vi "tes assemble (fuzzy) edit.vi"() -> ()   [LabVIEW 2015]
uses:
  <vilib>/userdefined/High Color/IMAQdx.ctl
  <vilib>/Platform/TimedLoop/XDataNode/timing_clust.ctl
  <vilib>/Platform/TimedLoop/XDataNode/nitl_modes.ctl
  <vilib>/Platform/TimedLoop/XDataNode/wakeup.ctl
  <vilib>/FPGAPlugInAG/myRIO-1900/niLvFpga_Open_myRIO-1900.vi
  <vilib>/rvi/interface/common/dynamic/niFpgaDynamicAddResources.vi
  <vilib>/addons/Fuzzy Logic/FL Fuzzy Controller (MIMO).vi
  <vilib>/FPGAPlugInAG/Dynamic/niLvFpga_Run_Dynamic.vi
  <vilib>/Utility/error.llb/Error Cluster From Error Code.vi
  <vilib>/rvi/errors/niLvFpgaAdjustHostInterfaceError.vi
  <vilib>/FPGAPlugInAG/Dynamic/niLvFpga_Close_Dynamic.vi
  <vilib>/addons/control/pid/pid.llb/PID (DBL).vi
  <vilib>/Platform/TimedLoop/XDataNode/XDataNode.xnode
  <vilib>/rvi/interface/nirviOpenFPGA/nirviOpenFPGA.xnode
  C/Users/ASUS/Documents/LabVIEW Data/TA/FPGA Bitfiles/FPGAv2_FPGATarget2_Assemble3_FPMe1Auxq6o.lvbitx
  C/Users/ASUS/Documents/LabVIEW Data/Assemble.vi
  <vilib>/rvi/interface/nirviMethod/nirviMethod.xnode
  <vilib>/rvi/interface/nirviReadWriteControl/nirviReadWriteControl.xnode
  <vilib>/rvi/interface/nirviCloseFPGA/nirviCloseFPGA.xnode
  <vilib>/rvi/Arithmetic/AddSubMult/XNode/nirviSatArithmetic.xnode
  <vilib>/rvi/interface/Simulation/niFpgaSimulationCallBeginRW.vi
  <vilib>/Platform/TimedLoop/XDataNode/XDNodeRunTimeDep.lvlib
  <vilib>/vision/driver/NI_Vision_Acquisition_Software.lvlib
  <resource>/objmgr/imaqdx.rc
  <vilib>/addons/control/pid/NI_PID_pid.lvlib
  <vilib>/addons/Fuzzy Logic/NI_Fuzzy_Logic_API.lvlib
  NiFpgaLv.dll
  <vilib>/Instr/_visa.llb/VISA Configure Serial Port (Instr).vi
panel:
  out "Battery percentage":dbl(slide) scale=0.0..100.0
  in  "file path":path=path "c:/captue.jpg"
  out "Distance":dbl
  in  "Capture pict.":bool
  out "video modes":string
  in  "video mode":u32=20
  out "?":T1(plugin-control)
  in  "webcam":T2="cam0"
  out "k.kanan":dbl
  out "k.kiri":dbl
  out "x-y 2":dbl
  out "x+y 2":dbl
  out "percp. 2":dbl
  out "w 2":dbl
  out "percp.":dbl
  out "w":dbl
  out "Velo":i32
  out "Acce":i32
  in  "interval 2":u32=1000
  out "Vel":i32
  out "Acc":i32
  in  "interval":u32=1000
  out "x-y":dbl
  out "x+y":dbl
  out "b":dbl
  out "a":dbl
  out "x = y?":bool
  out "(hi.lo)":u16
  out "Velocity (Counts/Interval) 4":i32
  out "Velocity (Counts/Interval) 3":i32
  out "Velocity (Counts/Interval) 2":i32
  out "Velocity (Counts/Interval)":i32
  out "Acceleration (rps/s) 4":dbl
  out "Acceleration (rps/s) 3":dbl
  out "Acceleration (rps/s) 2":dbl
  out "Acceleration (rps/s)":dbl
  out "frame rate [fps]":dbl
  out "STOP Indicator":bool
  in  "Run/Stop":bool
  out "RC ch3":u32
  out "heading":dbl
  in  "gyro reset":bool=TRUE
  out "heading error":dbl
  out "target bearing":dbl
  out "target distance":dbl
  in  "y target":dbl
  in  "x target":dbl
  out "Acceleration (x)[m/s^2] 2":dbl
  out "Speed (x) [m/s]":dbl
  out "(x) Accelero":dbl
  out "Acceleration (y)[m/s^2]  2":dbl
  out "Speed (y) [m/s]":dbl
  out "(y) Accelero":dbl
  out "Acceleration (z)[m/s^2]  2":dbl
  out "Speed (z) [m/s]":dbl
  out "(z) Accelero":dbl
  out "voltage":dbl
  out "var.RTH":dbl
  out "kec.kanan":dbl
  out "kec.kiri":dbl
  out "kecp.kanan":dbl
  out "kecp.kiri":dbl
  out "var.auto":dbl
  in  "Mode":bool
  in  "RTH":bool
  out "relay 4":bool
  out "relay 3":bool
  out "relay 2":bool
  out "relay1":bool
  out "bocor 2":bool
  out "Water_LVL2":dbl
  out "Water_LVL1":dbl
  out "bocor 1":bool
  out "Arus 4":dbl
  out "Arus 3":dbl
  out "Arus1":dbl
  out "Arus2":dbl
  out "En 8":bool
  out "En 7":bool
  out "En 6":bool
  out "En 5":bool
  out "En 4":bool
  out "En 3":bool
  out "En 2":bool
  out "En 1":bool
  out "Rpm 4":dbl
  out "Rpm 3":dbl
  out "Rpm 2":dbl
  out "Rpm 1":dbl
  out "To":dbl
  out "var. manual":dbl
  out "enc 4":i32
  out "enc 3":i32
  out "enc 2":i32
  out "enc 1":i32
  out "Time On4":dbl format="%.2f"
  out "Time On3":dbl format="%.2f"
  out "Time On2":dbl
  out "y position":dbl
  out "x position":dbl
  out "angle":dbl
  out "Toff":dbl
  out "Time On1":dbl
  out "ultrasonik4":sgl
  out "ultrasonik3":sgl
  out "ultrasonik2":sgl
  out "ultrasonik1":sgl
  out "RC ch2":u32
  out "RC ch1":u32
  out "US 4":u32
  out "US3":u32
  out "US2":u32
  out "US1":u32
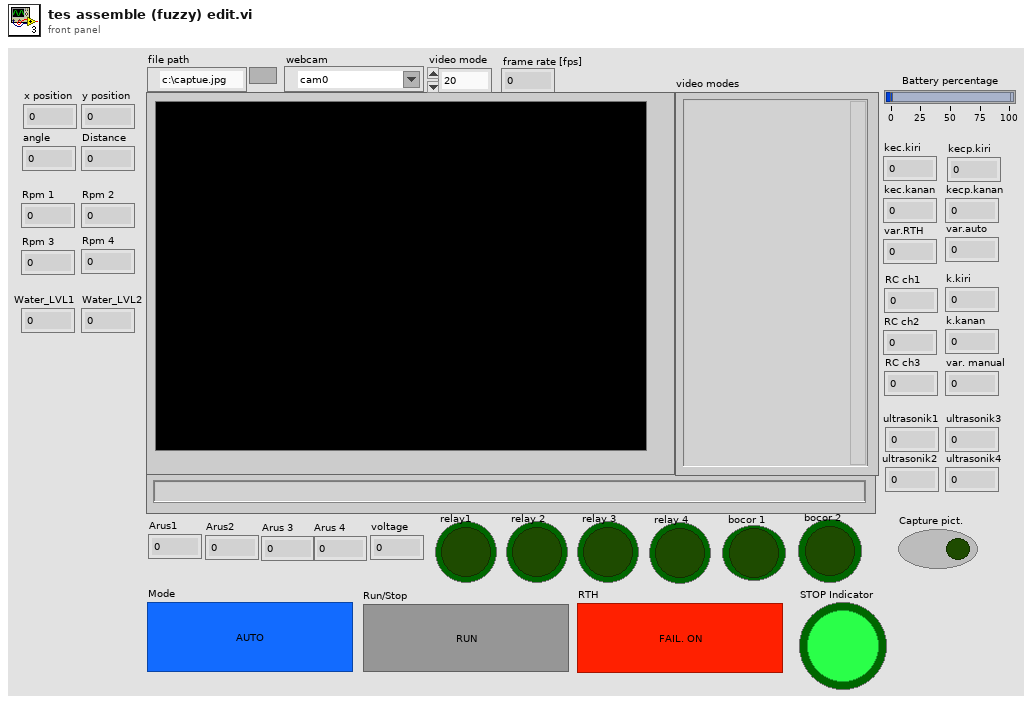
[diagram p1: front panel]
types:
  T1 = typedef "IMAQ Image.ctl" = refnum<image>
  T2 = typedef "IMAQdx.ctl" = refnum<k21>
  T3 = cluster{"Video Mode":u32, "Video Mode Name":string}[]
  T4 = typedef "XDNodeRunTimeDep.lvlib/timing_clust.ctl" = cluster{"Expected End [f-1]":u64, "Actual End [f-1]":u64, "Finished Late? [f-1]":bool, "Expected End [i-1]":u64, "Actual End [i-1]":u64, "Finished Late? [i-1]":bool, "Expected Start [i]":u64, "Actual Start [i]":u64, "Expected Start [f]":u64, "Actual Start [f]":u64, "Source Name":string, "Structure Name":string, "Period":i64, "Deadline":i64, "Offset":i64, "Start":i64, "Priority":i32, "Timeout":i32, "Mode":T5, "Wakeup Reason":T6, "Error":errorcluster, "Source Type":string, "Secondary Source Type":string, "Global End Time":u64, "Global Start Time":u64, "Frame Duration":u64, "Iteration Duration":u64, "Assigned CPU":i32, "I/O Scan Engine Mode":u32}
  T5 = typedef "XDNodeRunTimeDep.lvlib/nitl_modes.ctl" = enum32{"No Change", "Process missed periods, maintain original phase", "Discard missed periods, maintain original phase", "Process missed periods, ignore original phase", "Discard missed periods, ignore original phase"}
  T6 = typedef "XDNodeRunTimeDep.lvlib/wakeup.ctl" = enum32{"Normal", "Aborted", "Asynchronous wakeup", "Timing source error", "Timed loop error", "Timeout"}
  T7 = cluster{"proportional gain (Kc)":dbl, "integral time (Ti, min)":dbl, "derivative time (Td, min)":dbl}
  T8 = typedef "NI_Fuzzy_Logic_API.lvlib/FL System.ctl" = cluster{"input variables":T9[], "output variables":T9[], "rules":T12[], "defuzzification method":T18, "description":string, "user MF interpolating polynomials":T19[]}
  T9 = typedef "NI_Fuzzy_Logic_API.lvlib/FL Variable.ctl" = cluster{"name":string, "range":dbl[], "MFs":T10[]}
  T10 = typedef "NI_Fuzzy_Logic_API.lvlib/FL Membership Function.ctl" = cluster{"name":string, "shape":T11, "points":dbl[], "color":u32, "user-defined shape index":i32}
  T11 = typedef "NI_Fuzzy_Logic_API.lvlib/FL Membership Function Shape.ctl" = u16
  T12 = typedef "NI_Fuzzy_Logic_API.lvlib/FL Rule.ctl" = cluster{"antecedents":T13[], "antecedent connective":T15, "consequents":T16[], "consequent implication":T17, "degree of support":dbl}
  T13 = typedef "NI_Fuzzy_Logic_API.lvlib/FL Antecedent.ctl" = cluster{"Var Index":i32, "MF Index":i32, "Cond":T14}
  T14 = typedef "NI_Fuzzy_Logic_API.lvlib/FL Modifier.ctl" = u16
  T15 = typedef "NI_Fuzzy_Logic_API.lvlib/FL Antecedent Connective.ctl" = u16
  T16 = typedef "NI_Fuzzy_Logic_API.lvlib/FL Consequent.ctl" = cluster{"Var Index":i32, "MF Index":i32, "Cond":T14}
  T17 = typedef "NI_Fuzzy_Logic_API.lvlib/FL Consequent Implication.ctl" = u16
  T18 = typedef "NI_Fuzzy_Logic_API.lvlib/FL Defuzzification.ctl" = u16
  T19 = typedef "NI_Fuzzy_Logic_API.lvlib/FL Interpolating polynomials.ctl" = cluster{"X":dbl[], "Y":dbl[], "Y(x) coeff":dbl[][], "X(y) coeff":dbl[][], "Area(y) coeff":dbl[][], "coa_x(y) coeff":dbl[][]}
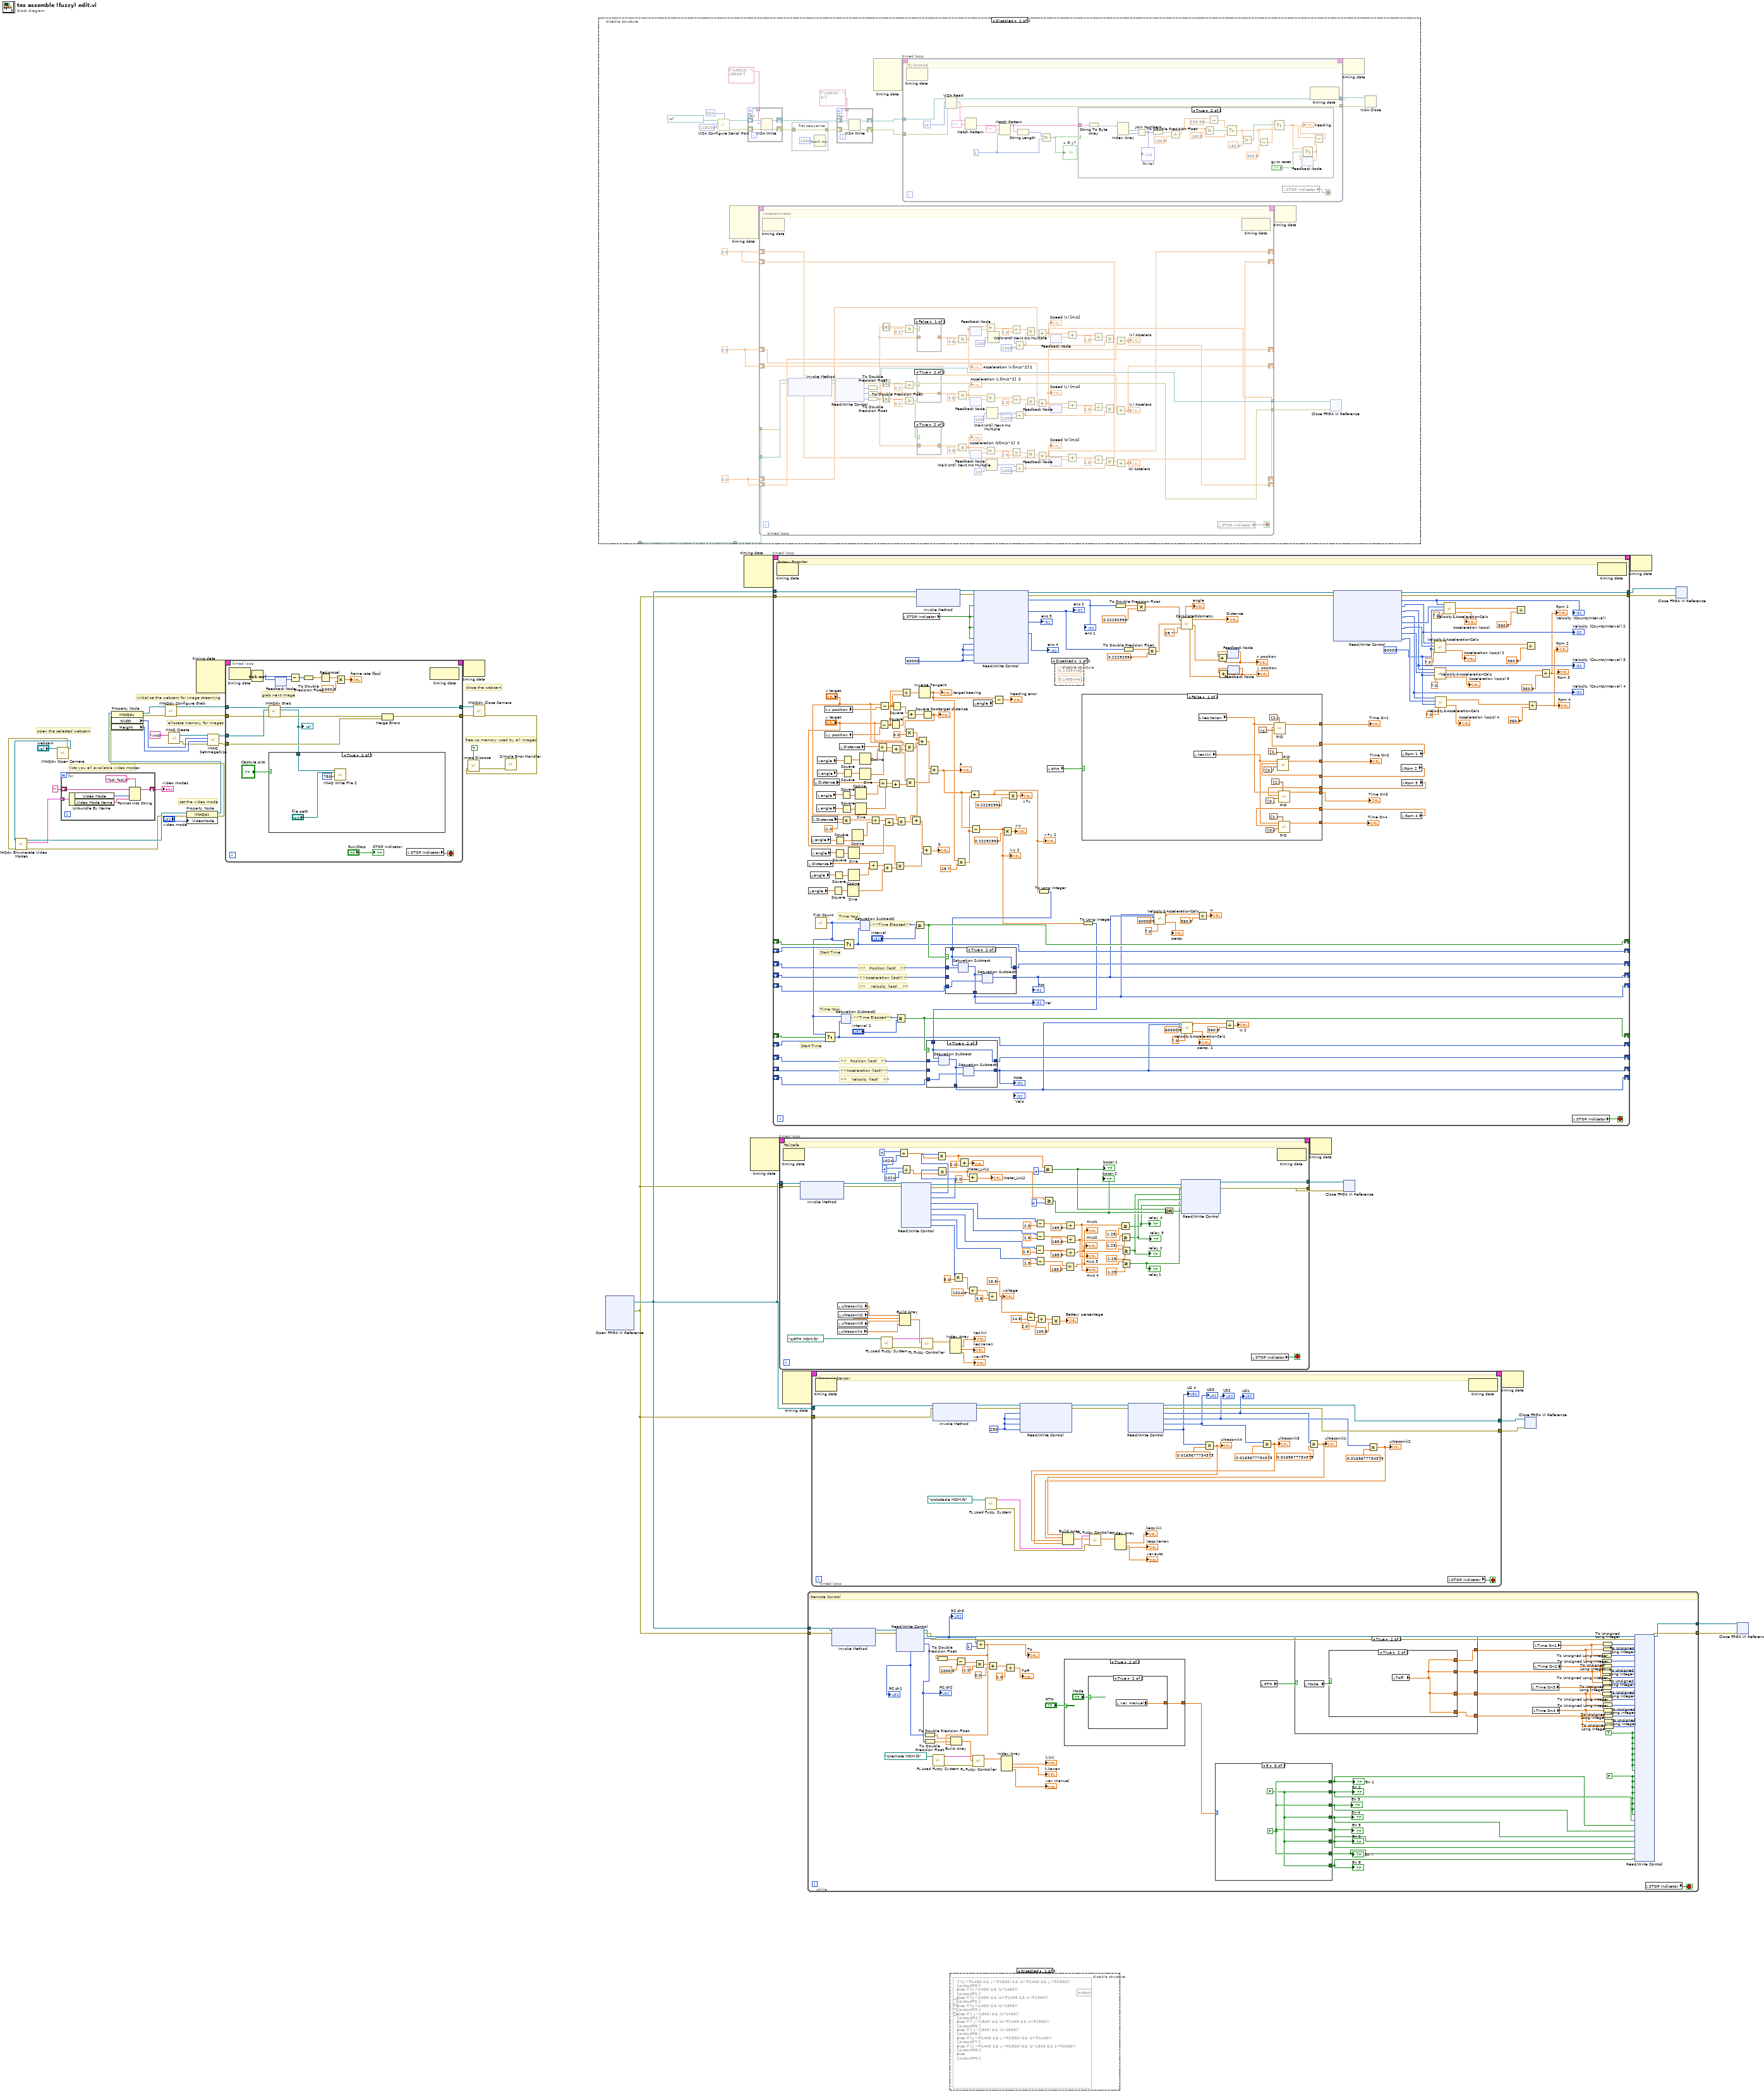
[diagram p0: block diagram]
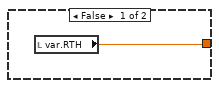
[diagram p4: hidden frame]
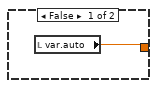
[diagram p5: hidden frame]
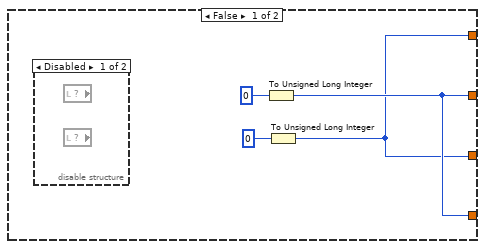
[diagram p6: hidden frame]
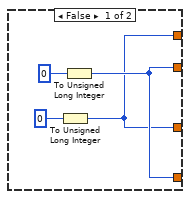
[diagram p8: hidden frame]
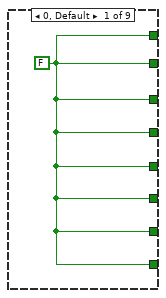
[diagram p9: hidden frame]
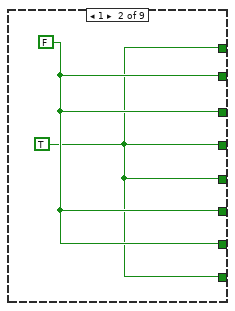
[diagram p10: hidden frame]
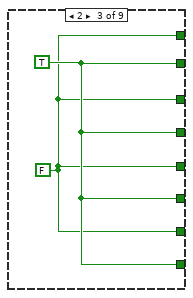
[diagram p11: hidden frame]
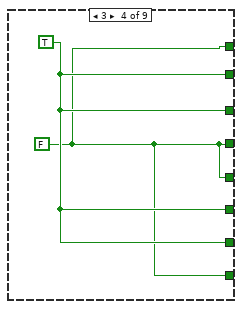
[diagram p12: hidden frame]
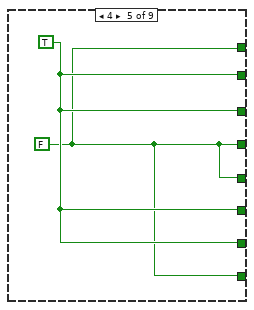
[diagram p13: hidden frame]
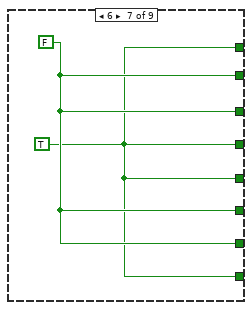
[diagram p14: hidden frame]
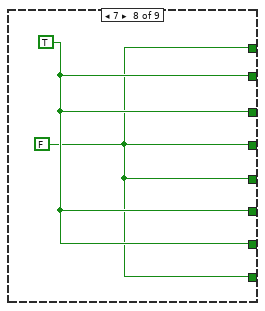
[diagram p15: hidden frame]
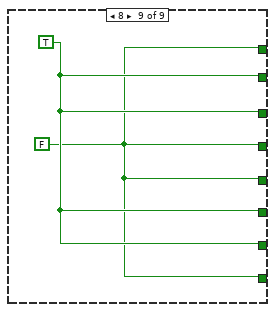
[diagram p16: hidden frame]
diagram:
  # "lists you all available video modes"
  # "close the webcam"
  # "open the selected webcam"
  # "set the video mode"
  # "allocate memory for images"
  # "initialize the webcam for image streaming"
  # "free up memory used by all images"
  n1 = call <vilib>:"IMAQdx Open Camera.vi"("Session In"="webcam") -> ("error out"=w5:errorcluster, "Session Out"=w6:T2)  [unwired: 2 in, 7 out]
  n2 = call <vilib>:"IMAQdx Enumerate Video Modes.vi"("error in"=w5, "Session In"=w6) -> ("error out"=w4:errorcluster, "Video Modes"=w9:T3, "Session Out"=w3:T2)  [unwired: 6 in, 1 out]
  n3 = for {
    tunnel: w9 -> [w51] mode=indexing
    shift-right: [w47] -> w8
    shift-left: "" -> [w46]
    n4 = Unbundle By Name(w51) -> ("Video Mode"=w49:u32, "Video Mode Name"=w48:string)
    n5 = Format Into String(format string="%d: %s\\n", initial string=w46, w49, w48) -> (resulting string=w47:string)  [unwired: 1 in, 1 out]
  }
  "video modes" <- w8
  n6 = call "IMAQ Create"("Image Name"="im0") -> ("New Image"=w19:T1, "error out"=w11:errorcluster)  [unwired: 3 in, 1 out]
  n7 = property on="Property Node" class="IMAQdx"(reference=w3, error in=w4, "VideoMode"="video mode") -> (reference out=w17:T2, error out=w14:errorcluster)
  n8 = property on="Property Node" class="IMAQdx"(reference=w17, error in=w14) -> (reference out=w16:T2, error out=w15:errorcluster, "Width"=w13:u32, "Height"=w12:u32)
  n9 = call <vilib>:"IMAQdx Configure Grab.vi"("error in"=w15, "Session In"=w16) -> ("error out"=w27:errorcluster, "Session Out"=w21:T2)  [unwired: 8 in]
  n10 = node-c288() -> (w2:T4)  [unwired: 4 in]
  n11 = call "IMAQ SetImageSize"("error in (no error)"=w11, "Y Resolution"=w12, "X Resolution"=w13, "Image"=w19) -> ("error out"=w10:errorcluster, "Image Out"=w18:T1)  [unwired: 1 in]
  n12 = timed-loop {
    tunnel: w18 -> [w69]
    tunnel: w27 -> [w67]
    tunnel: w21 -> [w68]
    tunnel: [w64] -> w24
    tunnel: [w65] -> w23
    tunnel: w10 -> [w54]
    timing: w2 -> [_]
    timing-out: [_] -> w1
    stop <- w62 stop-if-true
    # "grab next image"
    n13 = node-c288() -> ()  [unwired: 1 in, 1 out]
    n14 = Tick Count (ms)() -> (millisecond timer value=w61:u32)
    n15 = call <vilib>:"IMAQdx Grab.vi"("error in"=w67, "Image In"=w69, "Session In"=w68) -> ("error out"=w66:errorcluster, "Image Out"=w53:T1, "Session Out"=w65:T2)  [unwired: 5 in, 1 out]
    "?" <- w53
    n16 = case shown="True" "Capture pict." {
      tunnel: w53 -> [_ w72]
      frame False {
      }
      frame True {
        n17 = call-poly "IMAQ Write File 2"("Image Quality"=u32 750, "File Path"="file path", "Image"=w72) -> ()  [unwired: 7 in, 2 out]
      }
    }
    n18 = feedback #1() -> (w60:u32)  [unwired: 1 in]
    n19 = feedback-in #1(w61) -> ()
    n20 = Subtract(x=w61, y=w60) -> (x-y=w59:u32)
    n21 = To Double Precision Float(number=w59) -> (double precision float=w58:dbl)
    n22 = Reciprocal(x=w58) -> (1/x=w57:dbl)
    n23 = Multiply(x=w57, y=1000.0) -> (x*y=→"frame rate [fps]":dbl)
    n24 = Merge Errors(w66, w54) -> (w64:errorcluster)
    n25 = local read "STOP Indicator"() -> (w62:bool)
    n26 = node-c288() -> ()  [unwired: 1 in, 1 out]
    "STOP Indicator" <- "Run/Stop"
  }
  n27 = node-c288(w1) -> ()  [unwired: 1 out]
  n28 = call <vilib>:"IMAQdx Close Camera.vi"("error in"=w24, "Session In"=w23) -> ("error out"=w25:errorcluster)  [unwired: 9 out]
  n29 = call "Imaq Dispose"("All Images? (No)"=TRUE, "error in (no error)"=w25) -> ("error out"=w22:errorcluster)  [unwired: 4 in]
  n30 = call <vilib>:"Simple Error Handler.vi"("error in (no error)"=w22) -> ()  [unwired: 4 in, 5 out]
  n31 = disable-structure shown="Disabled" {
    disable-tunnel: _ -> [w90 _]
    disable-tunnel: _ -> [w89 _]
    frame Disabled {
      w91 = 0.0
      w92 = 0.0
      w93 = 0.0
      n32 = call-poly "VISA Configure Serial Port"("VISA resource name"=refnum<visa-resource-name> "ASRL1::INSTR", "termination char\n(0xA = '\\n' = LF)"=u8 104 ("termination char\n(0xA = '\\n' = LF)"), "baud rate (9600)"=u32 115200) -> ("VISA resource name out"=w87:refnum<visa-resource-name>, "error out"=w85:errorcluster)  [unwired: 11 in]
      n33 = node-c288() -> (w99:T4)  [unwired: 4 in]
      n34 = for {
        shift-right: [w110] -> w81
        shift-left: w87 -> [w111]
        tunnel: string[] ["\u001c", "\u0010"] -> [w109] mode=indexing
        shift-right: [w107] -> w78
        shift-left: w85 -> [w108]
        n35 = VISA Write(VISA resource name=w111, write buffer=w109, error in (no error)=w108) -> (VISA resource name out=w110:refnum<visa-resource-name>, error out=w107:errorcluster)  [unwired: 1 out]
      }
      n36 = timed-loop {
        timing: w99 -> [_]
        timing-out: [_] -> w98
        tunnel: [w234] -> w95
        tunnel: [w233] -> w94
        tunnel: w90 -> [w232]
        tunnel: w89 -> [w231]
        shift-right: [w208] -> _
        shift-left: w93 -> [w218]
        shift-right: [w158] -> _
        shift-left: w93 -> [w209]
        shift-right: [w185] -> _
        shift-left: w92 -> [w189]
        shift-right: [w157] -> _
        shift-left: w92 -> [w188]
        shift-right: [w160] -> _
        shift-left: w91 -> [w164]
        shift-right: [w159] -> _
        shift-left: w91 -> [w163]
        stop <- w156 stop-if-true
        # "Accelerometer"
        n37 = node-c288() -> ()  [unwired: 1 in, 1 out]
        n38 = xnode "Invoke Method"("FPGA VI Reference In"=w232, "error in"=w231) -> ("FPGA VI Reference Out"=w236:refnum<k20>, "error out"=w235:errorcluster)  [unwired: 1 in]
        n39 = xnode "Read/Write Control"("FPGA VI Reference In"=w236, "error in"=w235) -> ("FPGA VI Reference Out"=w234:refnum<k20>, "error out"=w233:errorcluster, "ACC.X.VAL"=w227:u16, "ACC.Y.VAL"=w187:u16, "ACC.Z.VAL"=w162:u16)
        n40 = To Double Precision Float(number=w227) -> (double precision float=w228:dbl)
        n41 = To Double Precision Float(number=w187) -> (double precision float=w186:dbl)
        n42 = To Double Precision Float(number=w162) -> (double precision float=w161:dbl)
        n43 = Absolute Value(x=w228) -> (abs(x)=w229:dbl)
        n44 = Absolute Value(x=w186) -> (abs(x)=w206:dbl)
        n45 = Absolute Value(x=w161) -> (abs(x)=w182:dbl)
        n46 = Greater?(x=w229, y=0.2) -> (0:w230:bool)
        n47 = Greater?(x=w206, y=0.2) -> (0:w207:bool)
        n48 = Greater?(x=w182, y=0.2) -> (0:w183:bool)
        n49 = case shown="False" w230 {
          tunnel: w228 -> [_ w239]
          tunnel: [_ w239] -> w225
          frame False {
          }
          frame True {
          }
        }
        n50 = case shown="True" w207 {
          tunnel: w186 -> [_ w238]
          tunnel: [_ w238] -> w184
          frame False {
          }
          frame True {
          }
        }
        n51 = case shown="True" w183 {
          tunnel: w161 -> [_ w237]
          tunnel: [_ w237] -> w180
          frame False {
          }
          frame True {
          }
        }
        n52 = Multiply(x=w225, y=9.8) -> (x*y=w216:dbl)
        "Acceleration (x)[m/s^2] 2" <- w216
        n53 = Multiply(x=w184, y=9.8) -> (x*y=w196:dbl)
        "Acceleration (y)[m/s^2]  2" <- w196
        n54 = Multiply(x=w180, y=9.8) -> (x*y=w171:dbl)
        "Acceleration (z)[m/s^2]  2" <- w171
        n55 = feedback-in #2(w216) -> ()
        n56 = feedback #2() -> (w217:dbl)  [unwired: 1 in]
        n57 = feedback #3() -> (w197:dbl)  [unwired: 1 in]
        n58 = feedback-in #3(w196) -> ()
        n59 = feedback #4() -> (w172:dbl)  [unwired: 1 in]
        n60 = feedback-in #4(w171) -> ()
        n61 = Add(x=w216, y=w217) -> (x+y=w223:dbl)
        n62 = Add(x=w196, y=w197) -> (x+y=w203:dbl)
        n63 = Add(x=w171, y=w172) -> (x+y=w178:dbl)
        n64 = Wait Until Next ms Multiple(millisecond multiple=10) -> (millisecond timer value=w152:u32)
        n65 = Wait Until Next ms Multiple(millisecond multiple=100) -> (millisecond timer value=w153:u32)
        n66 = Wait Until Next ms Multiple(millisecond multiple=100) -> (millisecond timer value=w154:u32)
        n67 = Divide(x=w223, y=2.0) -> (x/y=w222:dbl)
        n68 = Divide(x=w203, y=2.0) -> (x/y=w202:dbl)
        n69 = Divide(x=w178, y=2.0) -> (x/y=w177:dbl)
        n70 = Divide(x=w154, y=1000) -> (x/y=w211:dbl)
        n71 = Divide(x=w153, y=1000) -> (x/y=w191:dbl)
        n72 = Divide(x=w152, y=1000) -> (x/y=w166:dbl)
        n73 = Multiply(x=w222, y=w211) -> (x*y=w219:dbl)
        n74 = Multiply(x=w202, y=w191) -> (x*y=w198:dbl)
        n75 = Multiply(x=w177, y=w166) -> (x*y=w173:dbl)
        n76 = Add(x=w219, y=w218) -> (x+y=w208:dbl)
        "Speed (x) [m/s]" <- w208
        n77 = Add(x=w198, y=w189) -> (x+y=w185:dbl)
        "Speed (y) [m/s]" <- w185
        n78 = Add(x=w173, y=w164) -> (x+y=w160:dbl)
        "Speed (z) [m/s]" <- w160
        n79 = feedback #5() -> (w215:dbl)  [unwired: 1 in]
        n80 = feedback-in #5(w208) -> ()
        n81 = feedback #6() -> (w195:dbl)  [unwired: 1 in]
        n82 = feedback-in #6(w185) -> ()
        n83 = feedback #7() -> (w170:dbl)  [unwired: 1 in]
        n84 = feedback-in #7(w160) -> ()
        n85 = Add(x=w208, y=w215) -> (x+y=w214:dbl)
        n86 = Add(x=w185, y=w195) -> (x+y=w194:dbl)
        n87 = Add(x=w160, y=w170) -> (x+y=w169:dbl)
        n88 = Divide(x=w214, y=2.0) -> (x/y=w212:dbl)
        n89 = Divide(x=w194, y=2.0) -> (x/y=w192:dbl)
        n90 = Divide(x=w169, y=2.0) -> (x/y=w167:dbl)
        n91 = Multiply(x=w212, y=w211) -> (x*y=w210:dbl)
        n92 = Multiply(x=w192, y=w191) -> (x*y=w190:dbl)
        n93 = Multiply(x=w167, y=w166) -> (x*y=w165:dbl)
        n94 = Add(x=w210, y=w209) -> (x+y=w158:dbl)
        "(x) Accelero" <- w158
        n95 = Add(x=w190, y=w188) -> (x+y=w157:dbl)
        "(y) Accelero" <- w157
        n96 = Add(x=w165, y=w163) -> (x+y=w159:dbl)
        "(z) Accelero" <- w159
        n97 = local read "STOP Indicator"() -> (w156:bool)
        n98 = node-c288() -> ()  [unwired: 1 in, 1 out]
      }
      n99 = flat-sequence {
        tunnel: [w101] -> w79
        tunnel: w78 -> [w101]
        frame #0 {
          n100 = Wait (ms)(milliseconds to wait=u32 1000) -> ()  [unwired: 1 out]
        }
      }
      n101 = for {
        shift-right: [w105] -> w82
        shift-left: w81 -> [w106]
        tunnel: string[] ["\u001b", "\b"] -> [w104] mode=indexing
        shift-right: [w103] -> w83
        shift-left: w79 -> [w102]
        n102 = VISA Write(VISA resource name=w106, write buffer=w104, error in (no error)=w102) -> (VISA resource name out=w105:refnum<visa-resource-name>, error out=w103:errorcluster)  [unwired: 1 out]
      }
      n103 = node-c288() -> (w97:T4)  [unwired: 4 in]
      n104 = timed-loop {
        tunnel: w83 -> [w124]
        tunnel: w82 -> [w125]
        tunnel: [w114] -> w76
        tunnel: [w113] -> w75
        timing: w97 -> [_]
        timing-out: [_] -> w96
        stop <- w112 stop-if-true
        w117 = 1 ("offset (0)")
        # "Gyroscope"
        n105 = node-c288() -> ()  [unwired: 1 in, 1 out]
        n106 = VISA Read(VISA resource name=w125, byte count=u32 14, error in (no error)=w124) -> (VISA resource name out=w114:refnum<visa-resource-name>, read buffer=w122:string, error out=w113:errorcluster)  [unwired: 1 out]
        n107 = Match Pattern(string=w122, regular expression=";") -> (after substring=w120:string)  [unwired: 1 in, 3 out]
        n108 = Match Pattern(string=w120, regular expression=";", offset (0)=w117) -> (before substring=w115:string)  [unwired: 3 out]
        n109 = String Length(string=w115) -> (length=w118:i32)
        n110 = Equal?(x=w118, y=w117) -> (x = y?=w116:bool)
        "x = y?" <- w116
        n111 = case shown="True" w116 {
          tunnel: w115 -> [_ w149]
          frame False {
          }
          frame True {
            n112 = String To Byte Array(string=w149) -> (unsigned byte array=w148:u8[])
            n113 = Index Array(array=w148) -> (element #1=w147:u8, element #2=w146:u8)  [unwired: 2 in]
            n114 = Join Numbers(hi=w147, lo=w146) -> ((hi.lo)=w145:u16)
            "(hi.lo)" <- w145
            n115 = To Double Precision Float(number=w145) -> (double precision float=w144:dbl)
            n116 = Divide(x=w144, y=100.0) -> (x/y=w139:dbl)
            n117 = Greater?(x=w139, y=180.0) -> (0:w142:bool)
            n118 = Subtract(x=w139, y=295.35) -> (x-y=w140:dbl)
            n119 = Select(t=w140, s=w142, f=w139) -> (s? t:f=w134:dbl)
            n120 = Greater?(x=w134, y=180.0) -> (0:w136:bool)
            n121 = Subtract(x=w134, y=360.0) -> (x-y=w135:dbl)
            n122 = Select(t=w135, s=w136, f=w134) -> (s? t:f=w129:dbl)
            n123 = feedback #8() -> (w131:dbl)  [unwired: 1 in]
            n124 = Select(t=w129, s="gyro reset", f=w131) -> (s? t:f=w130:dbl)
            n125 = feedback-in #8(w130) -> ()
            n126 = Subtract(x=w129, y=w130) -> (x-y=→"heading":dbl)
          }
        }
        n127 = local read "STOP Indicator"() -> (w112:bool)
        n128 = node-c288() -> ()  [unwired: 1 in, 1 out]
      }
      n129 = node-c288(w98) -> ()  [unwired: 1 out]
      n130 = xnode "Close FPGA VI Reference"("FPGA VI Reference In"=w95, "error in"=w94) -> ()  [unwired: 1 out]
      n131 = node-c288(w96) -> ()  [unwired: 1 out]
      n132 = VISA Close(VISA resource name=w76, error in (no error)=w75) -> ()  [unwired: 1 out]
    }
    frame Enabled {
    }
  }
  n133 = xnode "Open FPGA VI Reference"() -> ("FPGA VI Reference Out"=w31:refnum<k20>, "error out"=w30:errorcluster)  [unwired: 2 in]
  n134 = node-c288() -> (w39:T4)  [unwired: 4 in]
  n135 = node-c288() -> (w35:T4)  [unwired: 4 in]
  n136 = timed-loop {
    timing: w39 -> [_]
    timing-out: [_] -> w38
    tunnel: w31 -> [w416]
    tunnel: w30 -> [w415]
    tunnel: [w409] -> w37
    tunnel: [w408] -> w36
    shift-right: [w302] -> _
    shift-left: _ -> [w307]
    shift-right: [w301] -> _
    shift-left: _ -> [w306]
    shift-right: [w300] -> _
    shift-left: _ -> [w305]
    shift-right: [w277] -> _
    shift-left: _ -> [w304]
    shift-right: [w278] -> _
    shift-left: _ -> [w303]
    shift-right: [w289] -> _
    shift-left: _ -> [w290]
    shift-right: [w288] -> _
    shift-left: _ -> [w291]
    shift-right: [w287] -> _
    shift-left: _ -> [w292]
    shift-right: [w269] -> _
    shift-left: _ -> [w293]
    shift-right: [w270] -> _
    shift-left: _ -> [w294]
    stop <- w414 stop-if-true
    w372 = u32 60000 ("Velocity Interval (uSec) 4")
    w373 = u32 60000 ("Velocity Interval (uSec) 4")
    # ">>Acceleration (last)>>"
    # "Start Time"
    # ">>    Velocity (last)    >>"
    # ">>   Position (last)   >>"
    # "Time Now"
    # ">>Time Elapsed>>"
    # ">>Acceleration (last)>>"
    # "Start Time"
    # ">>    Velocity (last)    >>"
    # ">>   Position (last)   >>"
    # "Time Now"
    # ">>Time Elapsed>>"
    # "Rotary Encoder"
    n137 = node-c288() -> ()  [unwired: 1 in, 1 out]
    n138 = local read "Distance"() -> (w257:dbl)
    n139 = local read "angle"() -> (w325:dbl)
    n140 = local read "angle"() -> (w330:dbl)
    n141 = local read "angle"() -> (w339:dbl)
    n142 = local read "angle"() -> (w335:dbl)
    n143 = local read "Distance"() -> (w258:dbl)
    n144 = local read "Distance"() -> (w259:dbl)
    n145 = call "Tick Count"() -> ("Tick Count(uSec)"=w295:u32)
    n146 = local read "angle"() -> (w356:dbl)
    n147 = local read "angle"() -> (w352:dbl)
    n148 = local read "angle"() -> (w363:dbl)
    n149 = local read "angle"() -> (w360:dbl)
    n150 = Select(t=w295, s=w290, f=w291) -> (s? t:f=w288:u32)
    n151 = local read "x position"() -> (w398:dbl)
    n152 = local read "y position"() -> (w397:dbl)
    n153 = Square(x=w325) -> (x^2=w326:dbl)
    n154 = Square(x=w330) -> (x^2=w329:dbl)
    n155 = Square(x=w335) -> (x^2=w336:dbl)
    n156 = Square(x=w339) -> (x^2=w340:dbl)
    n157 = local read "Distance"() -> (w260:dbl)
    n158 = Square(x=w356) -> (x^2=w355:dbl)
    n159 = Multiply(x=w258, y=-1.0) -> (x*y=w341:dbl)
    n160 = Square(x=w352) -> (x^2=w351:dbl)
    n161 = xnode ("Saturation Subtract2")("x"=w295, "y"=w288) -> ("x-y"=w296:u32)
    n162 = Square(x=w363) -> (x^2=w362:dbl)
    n163 = Square(x=w360) -> (x^2=w359:dbl)
    n164 = Select(t=w295, s=w307, f=w306) -> (s? t:f=w301:u32)
    n165 = Sine(x=w326) -> (sin(x)=w327:dbl)
    n166 = Cosine(x=w329) -> (cos(x)=w328:dbl)
    n167 = Sine(x=w336) -> (sin(x)=w334:dbl)
    n168 = Cosine(x=w340) -> (cos(x)=w338:dbl)
    n169 = Cosine(x=w355) -> (cos(x)=w354:dbl)
    n170 = Sine(x=w351) -> (sin(x)=w350:dbl)
    n171 = Cosine(x=w362) -> (cos(x)=w361:dbl)
    n172 = Sine(x=w359) -> (sin(x)=w358:dbl)
    n173 = xnode ("Saturation Subtract2")("x"=w295, "y"=w301) -> ("x-y"=w308:u32)
    n174 = Divide(x=w257, y=w328) -> (x/y=w331:dbl)
    n175 = Divide(x=w341, y=w338) -> (x/y=w337:dbl)
    n176 = Divide(x=w260, y=w361) -> (x/y=w357:dbl)
    n177 = Divide(x=w259, y=w354) -> (x/y=w353:dbl)
    n178 = Subtract(x="y target", y=w397) -> (x-y=w396:dbl)
    n179 = Subtract(x="x target", y=w398) -> (x-y=w395:dbl)
    n180 = Add(x=w331, y=w327) -> (x+y=w324:dbl)
    n181 = Add(x=w337, y=w334) -> (x+y=w333:dbl)
    n182 = Square(x=w396) -> (x^2=w400:dbl)
    n183 = Add(x=w353, y=w350) -> (x+y=w348:dbl)
    n184 = Add(x=w357, y=w358) -> (x+y=w349:dbl)
    n185 = Square(x=w395) -> (x^2=w401:dbl)
    n186 = Multiply(x="y target", y=w324) -> (x*y=w319:dbl)
    n187 = Greater Or Equal?(x=w296, y="interval 2") -> (x >= y?=w289:bool)
    n188 = Multiply(x="x target", y=w333) -> (x*y=w322:dbl)
    n189 = Divide(x=w396, y=w395) -> (x/y=w394:dbl)
    n190 = local read "STOP Indicator"() -> (w265:bool)
    n191 = Multiply(x="x target", y=w349) -> (x*y=w345:dbl)
    n192 = Multiply(x="y target", y=w348) -> (x*y=w343:dbl)
    n193 = Add(x=w401, y=w400) -> (x+y=w399:dbl)
    n194 = Greater Or Equal?(x=w308, y="interval") -> (x >= y?=w302:bool)
    n195 = xnode "Invoke Method"("FPGA VI Reference In"=w416, "error in"=w415) -> ("FPGA VI Reference Out"=w418:refnum<k20>, "error out"=w417:errorcluster)  [unwired: 1 in]
    n196 = Inverse Tangent(1:w394) -> (0:w314:dbl)
    "target bearing" <- w314
    n197 = Square Root(x=w399) -> (sqrt(x)=w346:dbl)
    "target distance" <- w346
    n198 = Multiply(x=w346, y=0.0) -> (x*y=w321:dbl)
    n199 = Add(x=w321, y=w322) -> (x+y=w320:dbl)
    n200 = Add(x=w321, y=w345) -> (x+y=w344:dbl)
    n201 = Add(x=w320, y=w319) -> (x+y=→"b":dbl)
    n202 = Add(x=w344, y=w343) -> (x+y=w316:dbl)
    "a" <- w316
    n203 = Multiply(x=w314, y=25.7) -> (x*y=w315:dbl)
    n204 = Add(x=w316, y=w315) -> (x+y=w299:dbl)
    "x+y 2" <- w299
    n205 = Subtract(x=w316, y=w315) -> (x-y=w285:dbl)
    "x-y 2" <- w285
    n206 = local read "angle"() -> (w392:dbl)
    n207 = xnode "Read/Write Control"("FPGA VI Reference In"=w418, "error in"=w417, "Position Reset"=w265, "Position Reset 2"=w265, "Position Reset 3"=w265, "Position Reset 4"=w265, "Velocity Interval (uSec)"=w373, "Velocity Interval (uSec) 2"=w373, "Velocity Interval (uSec) 3"=w373, "Velocity Interval (uSec) 4"=w373) -> ("FPGA VI Reference Out"=w407:refnum<k20>, "error out"=w406:errorcluster, "Position 1"=w250:i32, "Position 2"=w249:i32, "Position 3"=→"enc 3":i32, "Position 4"=→"enc 4":i32)
    "enc 1" <- w250
    "enc 2" <- w249
    n208 = Subtract(x=w314, y=w392) -> (x-y=→"heading error":dbl)
    n209 = Multiply(x=w285, y=0.22292994) -> (x*y=→"x-y":dbl)
    n210 = Multiply(x=w299, y=0.22292994) -> (x*y=→"x+y":dbl)
    n211 = To Long Integer(number=w299) -> (32bit integer=w298:i32)
    n212 = case shown="True" w302 {
      tunnel: w298 -> [_ w486]
      tunnel: w305 -> [w483 w490]
      tunnel: [w485 w489] -> w278
      tunnel: w303 -> [w485 w488]
      tunnel: [w484 w487] -> w277
      tunnel: w304 -> [w484 _]
      tunnel: [w483 w486] -> w300
      frame False {
      }
      frame True {
        n213 = xnode ("Saturation Subtract")("x"=w486, "y"=w490) -> ("x-y"=w489:i32)
        n214 = xnode ("Saturation Subtract3")("x"=w489, "y"=w488) -> ("x-y"=w487:i32)
      }
    }
    "Acc" <- w277
    "Vel" <- w278
    n215 = local read "RTH"() -> (w402:bool)
    n216 = disable-structure shown="Disabled" {
      frame Disabled {
        (unwired) 0.14854461 ("y")
        (unwired) 0.14854461 ("y")
      }
      frame Enabled {
      }
    }
    n217 = To Long Integer(number=w285) -> (32bit integer=w286:i32)
    n218 = case shown="True" w289 {
      tunnel: w286 -> [_ w432]
      tunnel: w292 -> [w429 w436]
      tunnel: [w431 w435] -> w270
      tunnel: w294 -> [w431 w434]
      tunnel: [w430 w433] -> w269
      tunnel: w293 -> [w430 _]
      tunnel: [w429 w432] -> w287
      frame False {
      }
      frame True {
        n219 = xnode ("Saturation Subtract")("x"=w432, "y"=w436) -> ("x-y"=w435:i32)
        n220 = xnode ("Saturation Subtract3")("x"=w435, "y"=w434) -> ("x-y"=w433:i32)
      }
    }
    "Acce" <- w269
    n221 = To Double Precision Float(number=w250) -> (double precision float=w413:dbl)
    n222 = To Double Precision Float(number=w249) -> (double precision float=w412:dbl)
    n223 = Multiply(x=w413, y=0.22292994) -> (x*y=w264:dbl)
    n224 = Multiply(x=w412, y=0.22292994) -> (x*y=w263:dbl)
    n225 = call "Velocity&AccelerationCalc.vi"("Pulses/Revolution"=7.0 ("y"), "Fixed Time \nInterval (uSec)"=60000.0 ("Fixed Time \nInterval (uSec)"), "Acceleration (Counts/Interval)"=w277, "Velocity (Counts/Interval)"=w278) -> ("Acceleration (rps/s)"=→"percp.":dbl, "Velocity (RPM)"=w281:dbl)
    n226 = call "CalculateOdometry.vi"("Left Wheel Distance"=w264, "Right Wheel Distance"=w263, "Wheel Base"=25.7) -> ("output variable"=→"angle":dbl, "Distance"=→"Distance":dbl, "X"=w252:dbl, "Y"=w251:dbl)  [unwired: 2 out]
    n227 = call "Velocity&AccelerationCalc.vi"("Pulses/Revolution"=7.0 ("y"), "Fixed Time \nInterval (uSec)"=60000.0 ("Fixed Time \nInterval (uSec)"), "Acceleration (Counts/Interval)"=w269, "Velocity (Counts/Interval)"=w270) -> ("Acceleration (rps/s)"=→"percp. 2":dbl, "Velocity (RPM)"=w273:dbl)
    n228 = Divide(x=w281, y=360.0) -> (x/y=→"w":dbl)
    n229 = Divide(x=w273, y=360.0) -> (x/y=→"w 2":dbl)
    n230 = feedback #9() -> (w255:dbl)  [unwired: 1 in]
    n231 = Add(x=w255, y=w252) -> (x+y=w254:dbl)
    "x position" <- w254
    n232 = feedback-in #9(w254) -> ()
    n233 = feedback #10() -> (w256:dbl)  [unwired: 1 in]
    n234 = Add(x=w256, y=w251) -> (x+y=w253:dbl)
    "y position" <- w253
    n235 = feedback-in #10(w253) -> ()
    n236 = xnode "Read/Write Control"("FPGA VI Reference In"=w407, "error in"=w406) -> ("FPGA VI Reference Out"=w409:refnum<k20>, "error out"=w408:errorcluster, "Velocity (Counts/Interval)"=w267:i32, "Velocity (Counts/Interval) 2"=w383:i32, "Velocity (Counts/Interval) 3"=w382:i32, "Velocity (Counts/Interval) 4"=w381:i32, "Acceleration (Counts/Interval)"=w391:i32, "Acceleration (Counts/Interval) 2"=w389:i32, "Acceleration (Counts/Interval) 3"=w388:i32, "Acceleration (Counts/Interval) 4"=w387:i32)
    "Velocity (Counts/Interval)" <- w267
    "Velocity (Counts/Interval) 2" <- w383
    "Velocity (Counts/Interval) 3" <- w382
    "Velocity (Counts/Interval) 4" <- w381
    n237 = local read "Rpm 2"() -> (w374:dbl)
    n238 = local read "Rpm 4"() -> (w376:dbl)
    n239 = local read "Rpm 1"() -> (w266:dbl)
    n240 = local read "Rpm 3"() -> (w375:dbl)
    n241 = case shown="False" w402 {
      tunnel: w266 -> [w535 w560]
      tunnel: [w536 w559] -> w268
      tunnel: [w534 w556] -> w405
      tunnel: w374 -> [w533 w555]
      tunnel: w375 -> [w532 w552]
      tunnel: [w531 w551] -> w404
      tunnel: [w529 w548] -> w403
      tunnel: w376 -> [w530 w547]
      frame False {
        n242 = local read "kec.kiri"() -> (w528:dbl)
        n243 = local read "kec.kanan"() -> (w527:dbl)
        n244 = call-poly <vilib>:"PID.vi"("output range"=cluster{"output high":dbl, "output low":dbl} {"output high"=2000.0, "output low"=0.0}, "PID gains"=T7 {"proportional gain (Kc)"=0.3, "integral time (Ti, min)"=0.75, "derivative time (Td, min)"=0.1875}, "process variable"=w535, "setpoint"=w527) -> ("output"=w536:dbl)  [unwired: 6 in, 1 out]
        n245 = call-poly <vilib>:"PID.vi"("output range"=cluster{"output high":dbl, "output low":dbl} {"output high"=2000.0, "output low"=0.0}, "PID gains"=T7 {"proportional gain (Kc)"=0.3, "integral time (Ti, min)"=0.75, "derivative time (Td, min)"=0.1875}, "process variable"=w533, "setpoint"=w528) -> ("output"=w534:dbl)  [unwired: 6 in, 1 out]
        n246 = call-poly <vilib>:"PID.vi"("output range"=cluster{"output high":dbl, "output low":dbl} {"output high"=2000.0, "output low"=0.0}, "PID gains"=T7 {"proportional gain (Kc)"=0.3, "integral time (Ti, min)"=0.75, "derivative time (Td, min)"=0.1875}, "process variable"=w532, "setpoint"=w527) -> ("output"=w531:dbl)  [unwired: 6 in, 1 out]
        n247 = call-poly <vilib>:"PID.vi"("output range"=cluster{"output high":dbl, "output low":dbl} {"output high"=2000.0, "output low"=0.0}, "PID gains"=T7 {"proportional gain (Kc)"=0.3, "integral time (Ti, min)"=0.75, "derivative time (Td, min)"=0.1875}, "process variable"=w530, "setpoint"=w528) -> ("output"=w529:dbl)  [unwired: 6 in, 1 out]
      }
      frame True {
        n248 = local read "Mode"() -> (w563:bool)
        n249 = case shown="False" w563 {
          tunnel: [w564 w566] -> w546
          tunnel: [w565 w567] -> w545
          frame False {
            n250 = local read "kecp.kanan"() -> (w565:dbl)
            n251 = local read "kecp.kiri"() -> (w564:dbl)
          }
          frame True {
            n252 = local read "k.kiri"() -> (w566:dbl)
            n253 = local read "k.kanan"() -> (w567:dbl)
          }
        }
        n254 = call-poly <vilib>:"PID.vi"("output range"=cluster{"output high":dbl, "output low":dbl} {"output high"=2000.0, "output low"=0.0}, "PID gains"=T7 {"proportional gain (Kc)"=0.3, "integral time (Ti, min)"=0.75, "derivative time (Td, min)"=0.1875}, "process variable"=w560, "setpoint"=w545) -> ("output"=w559:dbl)  [unwired: 6 in, 1 out]
        n255 = call-poly <vilib>:"PID.vi"("output range"=cluster{"output high":dbl, "output low":dbl} {"output high"=2000.0, "output low"=0.0}, "PID gains"=T7 {"proportional gain (Kc)"=0.3, "integral time (Ti, min)"=0.75, "derivative time (Td, min)"=0.1875}, "process variable"=w555, "setpoint"=w546) -> ("output"=w556:dbl)  [unwired: 6 in, 1 out]
        n256 = call-poly <vilib>:"PID.vi"("output range"=cluster{"output high":dbl, "output low":dbl} {"output high"=2000.0, "output low"=0.0}, "PID gains"=T7 {"proportional gain (Kc)"=0.3, "integral time (Ti, min)"=0.75, "derivative time (Td, min)"=0.1875}, "process variable"=w552, "setpoint"=w545) -> ("output"=w551:dbl)  [unwired: 6 in, 1 out]
        n257 = call-poly <vilib>:"PID.vi"("output range"=cluster{"output high":dbl, "output low":dbl} {"output high"=2000.0, "output low"=0.0}, "PID gains"=T7 {"proportional gain (Kc)"=0.3, "integral time (Ti, min)"=0.75, "derivative time (Td, min)"=0.1875}, "process variable"=w547, "setpoint"=w546) -> ("output"=w548:dbl)  [unwired: 6 in, 1 out]
      }
    }
    "Time On1" <- w268
    "Time On2" <- w405
    "Time On3" <- w404
    "Time On4" <- w403
    n258 = call "Velocity&AccelerationCalc.vi"("Pulses/Revolution"=7.0 ("y"), "Fixed Time \nInterval (uSec)"=w372, "Acceleration (Counts/Interval)"=w389, "Velocity (Counts/Interval)"=w383) -> ("Acceleration (rps/s)"=→"Acceleration (rps/s) 2":dbl, "Velocity (RPM)"=w368:dbl)
    n259 = call "Velocity&AccelerationCalc.vi"("Pulses/Revolution"=7.0 ("y"), "Fixed Time \nInterval (uSec)"=w372, "Acceleration (Counts/Interval)"=w388, "Velocity (Counts/Interval)"=w382) -> ("Acceleration (rps/s)"=→"Acceleration (rps/s) 3":dbl, "Velocity (RPM)"=w366:dbl)
    n260 = call "Velocity&AccelerationCalc.vi"("Pulses/Revolution"=7.0 ("y"), "Fixed Time \nInterval (uSec)"=w372, "Acceleration (Counts/Interval)"=w387, "Velocity (Counts/Interval)"=w381) -> ("Acceleration (rps/s)"=→"Acceleration (rps/s) 4":dbl, "Velocity (RPM)"=w364:dbl)
    n261 = call "Velocity&AccelerationCalc.vi"("Pulses/Revolution"=7.0 ("y"), "Fixed Time \nInterval (uSec)"=w372, "Acceleration (Counts/Interval)"=w391, "Velocity (Counts/Interval)"=w267) -> ("Acceleration (rps/s)"=→"Acceleration (rps/s)":dbl, "Velocity (RPM)"=w371:dbl)
    n262 = Divide(x=w371, y=360.0) -> ()  [unwired: 1 out]
    n263 = Divide(x=w368, y=360.0) -> ()  [unwired: 1 out]
    n264 = Divide(x=w364, y=360.0) -> (x/y=→"Rpm 2" →"Rpm 4":dbl)
    n265 = Divide(x=w366, y=360.0) -> (x/y=→"Rpm 1" →"Rpm 3":dbl)
    n266 = local read "STOP Indicator"() -> (w414:bool)
    n267 = node-c288() -> ()  [unwired: 1 in, 1 out]
  }
  n268 = timed-loop {
    timing: w35 -> [_]
    timing-out: [_] -> w34
    tunnel: w31 -> [w650]
    tunnel: w30 -> [w649]
    tunnel: [w644] -> w33
    tunnel: [w643] -> w32
    stop <- w642 stop-if-true
    w574 = 15.9 ("voltage")
    # "Failsafe"
    n269 = node-c288() -> ()  [unwired: 1 in, 1 out]
    n270 = xnode "Invoke Method"("FPGA VI Reference In"=w650, "error in"=w649) -> ("FPGA VI Reference Out"=w648:refnum<k20>, "error out"=w647:errorcluster)  [unwired: 1 in]
    n271 = local read "ultrasonik4"() -> (w631:sgl)
    n272 = local read "ultrasonik1"() -> (w628:sgl)
    n273 = local read "ultrasonik3"() -> (w630:sgl)
    n274 = local read "ultrasonik2"() -> (w629:sgl)
    n275 = call <vilib>:"FL Load Fuzzy System.vi"("file path"=path "c:/RTH MOM.fs") -> ("error out"=w626:errorcluster, "fuzzy system out"=w625:T8)  [unwired: 1 in, 8 out]
    n276 = Divide(x=u16 4 ("y"), y=u16 1024) -> (x/y=w613:dbl)
    n277 = Build Array(w628, w629, w630, w631) -> (w627:sgl[])
    n278 = Divide(x=u16 4 ("y"), y=u16 1024) -> (x/y=w614:dbl)
    n279 = xnode "Read/Write Control"("FPGA VI Reference In"=w648, "error in"=w647) -> ("FPGA VI Reference Out"=w646:refnum<k20>, "error out"=w645:errorcluster, "Water_LVL1"=w620:u16, "Water_LVL2"=w619:u16, "ACS712(1)"=w597:u16, "ACS712(2)"=w596:u16, "ACS712(3)"=w595:u16, "ACS712(4)"=w594:u16, "V sensor"=w634:u16)
    n280 = call-poly <vilib>:"FL Fuzzy Controller.vi"("error in (no error)"=w626, "input values"=w627, "fuzzy system in"=w625) -> ("output values"=w624:dbl[])  [unwired: 8 out]
    n281 = Multiply(x=w620, y=w613) -> (x*y=w593:dbl)
    n282 = Multiply(x=w619, y=w614) -> (x*y=w592:dbl)
    n283 = Index Array(array=w624) -> (element #1=→"kec.kiri":dbl, element #2=→"kec.kanan":dbl, element #3=→"var.RTH":dbl)  [unwired: 3 in]
    n284 = Multiply(x=w634, y=5.0) -> (x*y=w633:dbl)
    n285 = Add(x=w593, y=2.0) -> (x+y=→"Water_LVL1":dbl)
    n286 = Add(x=w592, y=2.0) -> (x+y=→"Water_LVL2":dbl)
    n287 = Divide(x=w633, y=1024.0) -> (x/y=w621:dbl)
    n288 = Divide(x=w621, y=0.8) -> ()  [unwired: 1 out]
    n289 = Subtract(x=w574, y=14.8) -> (x-y=w591:dbl)
    n290 = Subtract(x=w595, y=2.5) -> (x-y=w600:dbl)
    n291 = Subtract(x=w597, y=2.5) -> (x-y=w604:dbl)
    n292 = Subtract(x=w596, y=2.5) -> (x-y=w602:dbl)
    n293 = Subtract(x=w594, y=2.5) -> (x-y=w598:dbl)
    n294 = Divide(x=w591, y=2.0) -> (x/y=w589:dbl)
    n295 = Greater Or Equal?(x=w593, y=u16 4) -> (x >= y?=w582:bool)
    "bocor 1" <- w582
    n296 = Greater Or Equal?(x=w592, y=u16 4) -> (x >= y?=w581:bool)
    "bocor 2" <- w581
    n297 = Multiply(x=w589, y=100.0) -> (x*y=→"Battery percentage":dbl)
    n298 = Divide(x=w598, y=185.0) -> (x/y=w573:dbl)
    "Arus1" <- w573
    n299 = Divide(x=w604, y=185.0) -> (x/y=w570:dbl)
    "Arus 4" <- w570
    n300 = Divide(x=w600, y=185.0) -> (x/y=w572:dbl)
    "Arus2" <- w572
    n301 = Divide(x=w602, y=185.0) -> (x/y=w571:dbl)
    "Arus 3" <- w571
    n302 = Greater Or Equal?(x=w570, y=1.25) -> (x >= y?=w579:bool)
    "relay 4" <- w579
    n303 = Greater Or Equal?(x=w571, y=1.25) -> (x >= y?=w576:bool)
    "relay 3" <- w576
    n304 = Greater Or Equal?(x=w572, y=1.25) -> (x >= y?=w580:bool)
    "relay 2" <- w580
    n305 = Greater Or Equal?(x=w573, y=1.25) -> (x >= y?=w575:bool)
    "relay1" <- w575
    n306 = Or(x=w582, y=w581) -> (x .or. y?=w577:bool)
    n307 = xnode "Read/Write Control"("FPGA VI Reference In"=w646, "error in"=w645, "Relay Motor 1"=w575, "Relay motor 2"=w580, "Relay motor 3"=w576, "Relay motor 4"=w579, "Relay kebocoran"=w577) -> ("FPGA VI Reference Out"=w644:refnum<k20>, "error out"=w643:errorcluster)
    n308 = local read "STOP Indicator"() -> (w642:bool)
    n309 = node-c288() -> ()  [unwired: 1 in, 1 out]
    "voltage" <- w574
  }
  n310 = node-c288() -> (w43:T4)  [unwired: 4 in]
  n311 = while {
    tunnel: [w711] -> w45
    tunnel: [w709] -> w44
    tunnel: w31 -> [w721]
    tunnel: w30 -> [w720]
    stop <- w722 stop-if-true
    w682 = FALSE ("E2O")
    w683 = TRUE ("E2O")
    # "Remote Control"
    n312 = xnode "Invoke Method"("FPGA VI Reference In"=w721, "error in"=w720) -> ("FPGA VI Reference Out"=w719:refnum<k20>, "error out"=w718:errorcluster)  [unwired: 1 in]
    n313 = xnode "Read/Write Control"("FPGA VI Reference In"=w719, "error in"=w718) -> ("FPGA VI Reference Out"=w710:refnum<k20>, "error out"=w708:errorcluster, "Channel 3"=w663:u32, "Channel) 2"=w662:u32, "Channel 1"=w661:u32)
    "RC ch1" <- w661
    "RC ch2" <- w662
    "RC ch3" <- w663
    n314 = To Double Precision Float(number=w661) -> (double precision float=w671:dbl)
    n315 = To Double Precision Float(number=w662) -> (double precision float=w672:dbl)
    n316 = call <vilib>:"FL Load Fuzzy System.vi"("file path"=path "c:/remote MOM.fs") -> ("error out"=w675:errorcluster, "fuzzy system out"=w674:T8)  [unwired: 1 in, 8 out]
    n317 = Divide(x=w663, y=u32 1) -> (x/y=w664:dbl)
    "To" <- w664
    n318 = To Double Precision Float(number=w664) -> (double precision float=w712:dbl)
    n319 = Build Array(w671, w672, w664) -> (w670:dbl[])
    n320 = Subtract(x=w712, y=sgl 2000.0) -> (x-y=w717:dbl)
    n321 = call-poly <vilib>:"FL Fuzzy Controller.vi"("error in (no error)"=w675, "input values"=w670, "fuzzy system in"=w674) -> ("output values"=w673:dbl[])  [unwired: 8 out]
    n322 = Multiply(x=w717, y=sgl -1.0) -> (x*y=w716:dbl)
    n323 = Add(x=w716, y=sgl 0.0 ("-y")) -> (x+y=w701:dbl)
    n324 = Index Array(array=w673) -> (element #1=→"k.kiri":dbl, element #2=→"k.kanan":dbl, element #3=→"var. manual":dbl)  [unwired: 3 in]
    n325 = Divide(x=w701, y=1.0) -> (x/y=→"Toff":dbl)
    n326 = case shown="True" "RTH" {
      tunnel: [w723 w724] -> w676
      frame False {
        n327 = local read "var.RTH"() -> (w723:dbl)
      }
      frame True {
        n328 = case shown="True" "Mode" {
          tunnel: [w726 w727] -> w724
          frame False {
            n329 = local read "var.auto"() -> (w726:dbl)
          }
          frame True {
            n330 = local read "var. manual"() -> (w727:dbl)
          }
        }
      }
    }
    n331 = case shown="5" w676 {
      tunnel: [w742 w743 w745 w747 w749 w752 w753 w755 w757] -> w659
      tunnel: [w742 w744 w746 w748 w750 w751 w754 w756 w758] -> w660
      tunnel: [w742 w744 w745 w748 w750 w752 w754 w756 w758] -> w658
      tunnel: [w742 w743 w746 w747 w749 w751 w753 w755 w757] -> w657
      tunnel: [w742 w743 w745 w747 w749 w752 w753 w755 w757] -> w680
      tunnel: [w742 w744 w746 w748 w750 w751 w754 w756 w758] -> w681
      tunnel: [w742 w744 w745 w748 w750 w752 w754 w756 w758] -> w679
      tunnel: [w742 w743 w746 w747 w749 w751 w753 w755 w757] -> w678
      frame 0, Default {
        w742 = FALSE ("En")
      }
      frame 1 {
        w743 = TRUE ("En")
        w744 = FALSE ("En")
      }
      frame 2 {
        w745 = FALSE ("En")
        w746 = TRUE ("En")
      }
      frame 3 {
        w747 = FALSE ("En")
        w748 = TRUE ("En")
      }
      frame 4 {
        w749 = FALSE ("En")
        w750 = TRUE ("En")
      }
      frame 5 {
        w752 = TRUE ("En")
        w751 = FALSE ("En")
      }
      frame 6 {
        w753 = TRUE ("En")
        w754 = FALSE ("En")
      }
      frame 7 {
        w755 = FALSE ("En")
        w756 = TRUE ("En")
      }
      frame 8 {
        w757 = FALSE ("En")
        w758 = TRUE ("En")
      }
    }
    "En 1" <- w659
    "En 2" <- w660
    "En 3" <- w658
    "En 4" <- w657
    "En 5" <- w680
    "En 6" <- w681
    "En 7" <- w679
    "En 8" <- w678
    n332 = local read "RTH"() -> (w703:bool)
    n333 = case shown="True" w703 {
      tunnel: [w730 w735] -> w654
      tunnel: [w731 w734] -> w653
      tunnel: [w730 w733] -> w686
      tunnel: [w731 w732] -> w684
      frame False {
        n334 = disable-structure shown="Disabled" {
          frame Disabled {
            n335 = local read item#-1() -> ()  [unwired: 1 out]
            n336 = local read item#-1() -> ()  [unwired: 1 out]
          }
          frame Enabled {
          }
        }
        n337 = To Unsigned Long Integer(number=u32 0) -> (unsigned 32bit integer=w731:u32)
        n338 = To Unsigned Long Integer(number=u32 0) -> (unsigned 32bit integer=w730:u32)
      }
      frame True {
        n339 = local read "Mode"() -> (w736:bool)
        n340 = case shown="True" w736 {
          tunnel: [w739 w741] -> w735
          tunnel: [w740 w741] -> w734
          tunnel: [w739 w741] -> w733
          tunnel: [w740 w741] -> w732
          frame False {
            n341 = To Unsigned Long Integer(number=u32 0) -> (unsigned 32bit integer=w739:u32)
            n342 = To Unsigned Long Integer(number=u32 0) -> (unsigned 32bit integer=w740:u32)
          }
          frame True {
            n343 = local read "Toff"() -> (w741:dbl)
          }
        }
      }
    }
    n344 = local read "Time On3"() -> (w687:dbl)
    n345 = local read "Time On4"() -> (w685:dbl)
    n346 = local read "Time On1"() -> (w656:dbl)
    n347 = local read "Time On2"() -> (w655:dbl)
    n348 = To Unsigned Long Integer(number=w656) -> (unsigned 32bit integer=w706:u32)
    n349 = To Unsigned Long Integer(number=w653) -> (unsigned 32bit integer=w697:u32)
    n350 = To Unsigned Long Integer(number=w655) -> (unsigned 32bit integer=w704:u32)
    n351 = To Unsigned Long Integer(number=w653) -> (unsigned 32bit integer=w696:u32)
    n352 = To Unsigned Long Integer(number=w687) -> (unsigned 32bit integer=w695:u32)
    n353 = To Unsigned Long Integer(number=w654) -> (unsigned 32bit integer=w698:u32)
    n354 = To Unsigned Long Integer(number=w655) -> (unsigned 32bit integer=w705:u32)
    n355 = To Unsigned Long Integer(number=w686) -> (unsigned 32bit integer=w694:u32)
    n356 = To Unsigned Long Integer(number=w656) -> (unsigned 32bit integer=w707:u32)
    n357 = To Unsigned Long Integer(number=w654) -> (unsigned 32bit integer=w699:u32)
    n358 = To Unsigned Long Integer(number=w687) -> (unsigned 32bit integer=w693:u32)
    n359 = To Unsigned Long Integer(number=w686) -> (unsigned 32bit integer=w692:u32)
    n360 = To Unsigned Long Integer(number=w685) -> (unsigned 32bit integer=w691:u32)
    n361 = To Unsigned Long Integer(number=w684) -> (unsigned 32bit integer=w690:u32)
    n362 = To Unsigned Long Integer(number=w685) -> (unsigned 32bit integer=w689:u32)
    n363 = To Unsigned Long Integer(number=w684) -> (unsigned 32bit integer=w688:u32)
    n364 = xnode "Read/Write Control"("FPGA VI Reference In"=w710, "error in"=w708, "ton"=w707, "tof"=w699, "ton 2"=w706, "tof 2"=w698, "ton 3"=w705, "tof 3"=w697, "ton 4"=w704, "tof 4"=w696, "ton 5"=w695, "tof 5"=w694, "ton 6"=w693, "tof 6"=w692, "ton 7"=w691, "tof 7"=w690, "ton 8"=w689, "tof 8"=w688, "E1O"=w683, "E2O"=w683, "E3O"=w683, "E4O"=w683, "E5O"=w683, "E6O"=w683, "E7O"=w683, "E8O"=w683, "EI1"=w682, "EI2"=w682, "EI3"=w682, "EI4"=w682, "EI54"=w682, "EI6"=w682, "EI7"=w682, "EI8"=w682, "En1"=w660, "En2"=w659, "En3"=w658, "En4"=w657, "En5"=w681, "En6"=w680, "En7"=w679, "En8"=w678) -> ("FPGA VI Reference Out"=w711:refnum<k20>, "error out"=w709:errorcluster)
    n365 = local read "STOP Indicator"() -> (w722:bool)
  }
  n366 = timed-loop {
    timing: w43 -> [_]
    timing-out: [_] -> w42
    tunnel: [w785] -> w41
    tunnel: [w784] -> w40
    tunnel: w31 -> [w783]
    tunnel: w30 -> [w782]
    stop <- w788 stop-if-true
    w767 = u32 250 ("Trigger pulse interval 1")
    # "Ultrasonic Sensor"
    n367 = node-c288() -> ()  [unwired: 1 in, 1 out]
    n368 = xnode "Invoke Method"("FPGA VI Reference In"=w783, "error in"=w782) -> ("FPGA VI Reference Out"=w781:refnum<k20>, "error out"=w780:errorcluster)  [unwired: 1 in]
    n369 = call <vilib>:"FL Load Fuzzy System.vi"("file path"=path "c:/obstacle MOM.fs") -> ("error out"=w769:errorcluster, "fuzzy system out"=w770:T8)  [unwired: 1 in, 8 out]
    n370 = xnode "Read/Write Control"("FPGA VI Reference In"=w781, "error in"=w780, "Trigger pulse interval 1"=w767, "Trigger pulse interva 2"=w767, "Trigger pulse interval 3"=w767, "Trigger pulse interval 4"=w767) -> ("FPGA VI Reference Out"=w787:refnum<k20>, "error out"=w786:errorcluster)
    n371 = xnode "Read/Write Control"("FPGA VI Reference In"=w787, "error in"=w786) -> ("FPGA VI Reference Out"=w785:refnum<k20>, "error out"=w784:errorcluster, "time of flight 1"=w779:u32, "time of flight 2"=w778:u32, "time of flight 3"=w775:u32, "time of flight 4"=w773:u32)
    "US1" <- w779
    "US2" <- w778
    "US3" <- w775
    "US 4" <- w773
    n372 = Multiply(x=w773, y=sgl 0.016967773) -> (x*y=w765:sgl)
    "ultrasonik4" <- w765
    n373 = Multiply(x=w775, y=sgl 0.016967773) -> (x*y=w764:sgl)
    "ultrasonik3" <- w764
    n374 = Multiply(x=w779, y=sgl 0.016967773) -> (x*y=w763:sgl)
    "ultrasonik1" <- w763
    n375 = Multiply(x=w778, y=sgl 0.016967773) -> (x*y=w762:sgl)
    "ultrasonik2" <- w762
    n376 = Build Array(w763, w762, w764, w765) -> (w772:sgl[])
    n377 = call-poly <vilib>:"FL Fuzzy Controller.vi"("error in (no error)"=w769, "input values"=w772, "fuzzy system in"=w770) -> ("output values"=w771:dbl[])  [unwired: 8 out]
    n378 = Index Array(array=w771) -> (element #1=→"kecp.kiri":dbl, element #2=→"kecp.kanan":dbl, element #3=→"var.auto":dbl)  [unwired: 3 in]
    n379 = local read "STOP Indicator"() -> (w788:bool)
    n380 = node-c288() -> ()  [unwired: 1 in, 1 out]
  }
  n381 = disable-structure shown="Disabled" {
    frame Disabled {
      n382 = formula code="if ((y>=1400 && y<=1500) && (z>=1400 && y<=1500))\n{output=0;} \nelse if ((y<1400) && (z<1400))\n{output=1;}\nelse if ((y<1400) && (z>=1400 && z<=1500))\n{output=2;}\nelse if ((y<1400) && (z>1500))\n{output=3;}\nelse if (( y>1500) && (z<1400))\n{output=4;}\nelse if (( y>1500) && (z>=1400 && z<=1500))\n{output=5;}\nelse if (( y>1500) && (z>1500))\n{output=6;}\nelse if ((y>=1400 && y<=1500) && (z<=1400))\n{output=7;}\nelse if ((y>=1400 && y<=1500) && (z>1500 && z<=2000))\n{output=8;}\nelse\n{output=9;}"() -> ("output"=w791:dbl)  [unwired: 2 in]
    }
    frame Enabled {
    }
  }
  n383 = node-c288(w34) -> ()  [unwired: 1 out]
  n384 = xnode "Close FPGA VI Reference"("FPGA VI Reference In"=w33, "error in"=w32) -> ()  [unwired: 1 out]
  n385 = node-c288(w42) -> ()  [unwired: 1 out]
  n386 = xnode "Close FPGA VI Reference"("FPGA VI Reference In"=w41, "error in"=w40) -> ()  [unwired: 1 out]
  n387 = node-c288(w38) -> ()  [unwired: 1 out]
  n388 = xnode "Close FPGA VI Reference"("FPGA VI Reference In"=w37, "error in"=w36) -> ()  [unwired: 1 out]
  n389 = xnode "Close FPGA VI Reference"("FPGA VI Reference In"=w45, "error in"=w44) -> ()  [unwired: 1 out]
